vi "Module Identities.vi"(8 "error in (no error)":errorcluster, 11 "Hardware Info Module in":refnum<class "Hardware Info Module.lvclass">) -> (0 "error out":errorcluster, 2 "Identities":refnum<class "Identity.lvclass">[](array[class]), 3 "Hardware Info Module out":refnum<class "Hardware Info Module.lvclass">)   [LabVIEW 2020, in "Volatus.lvlib" / "Hardware Info Module.lvclass"]
uses:
  Hardware Info Module.lvclass
  Identity/Identity.lvclass
  Hardware Info Module.lvclass/Hardware Info Module.ctl
  Hardware Info Identity/Hardware Info Identity.lvclass
  C:/dev/lv20CE/relink/lv-volatus/Volatus/Hardware Info Identity/Hardware Info Identity.lvclass
  C:/dev/lv20CE/relink/lv-volatus/Volatus/Identity/Identity.lvclass
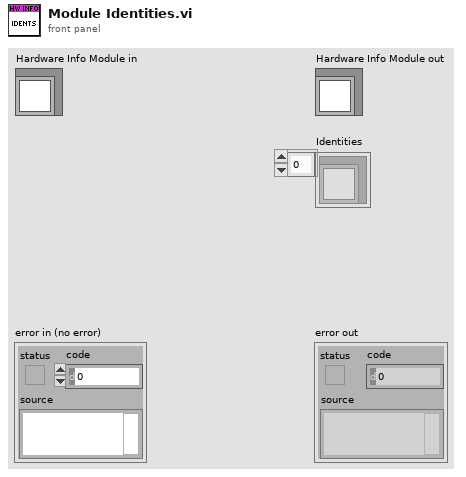
[diagram p1: front panel]
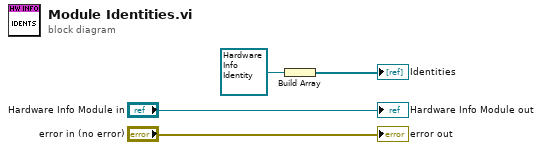
[diagram p0: block diagram]
diagram:
  n1 = Build Array(refnum<class "Hardware Info Identity.lvclass"> refnum ("Volatus:Hardware Info Identity.lvclass")) -> (→"Identities":refnum<class "Hardware Info Identity.lvclass">[])
  "error out" <- "error in (no error)"
  "Hardware Info Module out" <- "Hardware Info Module in"
